vi "Update Path.vi"(8 "error in (no error)":errorcluster, 10 "Active Test Executive Path":path, 11 "Test Executive Builder Active Path View in":refnum<class "Test Executive Builder Active Path View.lvclass">) -> (0 "error out":errorcluster, 3 "Test Executive Builder Active Path View out":refnum<class "Test Executive Builder Active Path View.lvclass">)   [LabVIEW 2017, in "Test Executive Builder Active Path View.lvclass"]
uses:
  <vilib>/gpm_packages/@cs/Test-executive-builder/Source/Active Path View/Test Executive Builder Active Path View/Test Executive Builder Active Path View.lvclass
  <vilib>/gpm_packages/@cs/Test-executive-builder/Source/Active Path View/Test Executive Builder Active Path View/Test Executive Builder Active Path View.lvclass/Test Executive Builder Active Path View.ctl
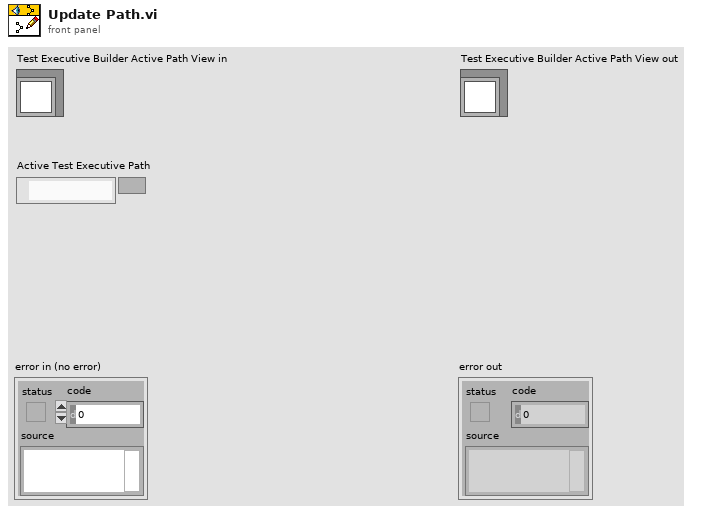
[diagram p1: front panel]
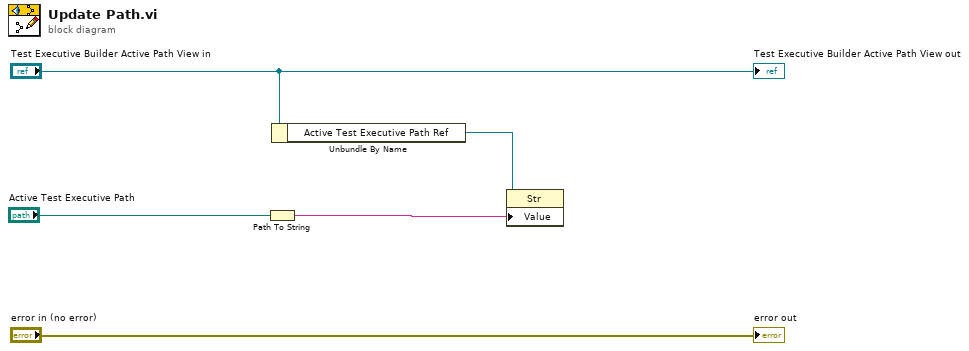
[diagram p0: block diagram]
diagram:
  n1 = Path To String(path="Active Test Executive Path") -> (string=w1:string)
  n2 = Unbundle By Name("Test Executive Builder Active Path View in") -> ("Active Test Executive Path Ref"=w2:refnum<vi>)
  n3 = property class="Str"(reference=w2, "Value"=w1) -> ()  [unwired: 1 in, 2 out]
  "error out" <- "error in (no error)"
  "Test Executive Builder Active Path View out" <- "Test Executive Builder Active Path View in"
